vi "Func_SpecificTagReferences.vi"(8 "error in (no error)":errorcluster, 10 "Paths Array":path[](array[path]), 11 "Data Type Name":string) -> (0 "error out":errorcluster)   [LabVIEW 2010, in "TemplateGenerator.lvlib"]
uses:
  TemplateGenerator.lvlib
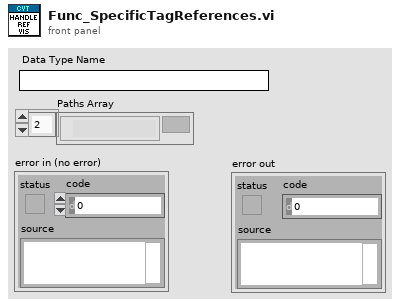
[diagram p1: front panel]
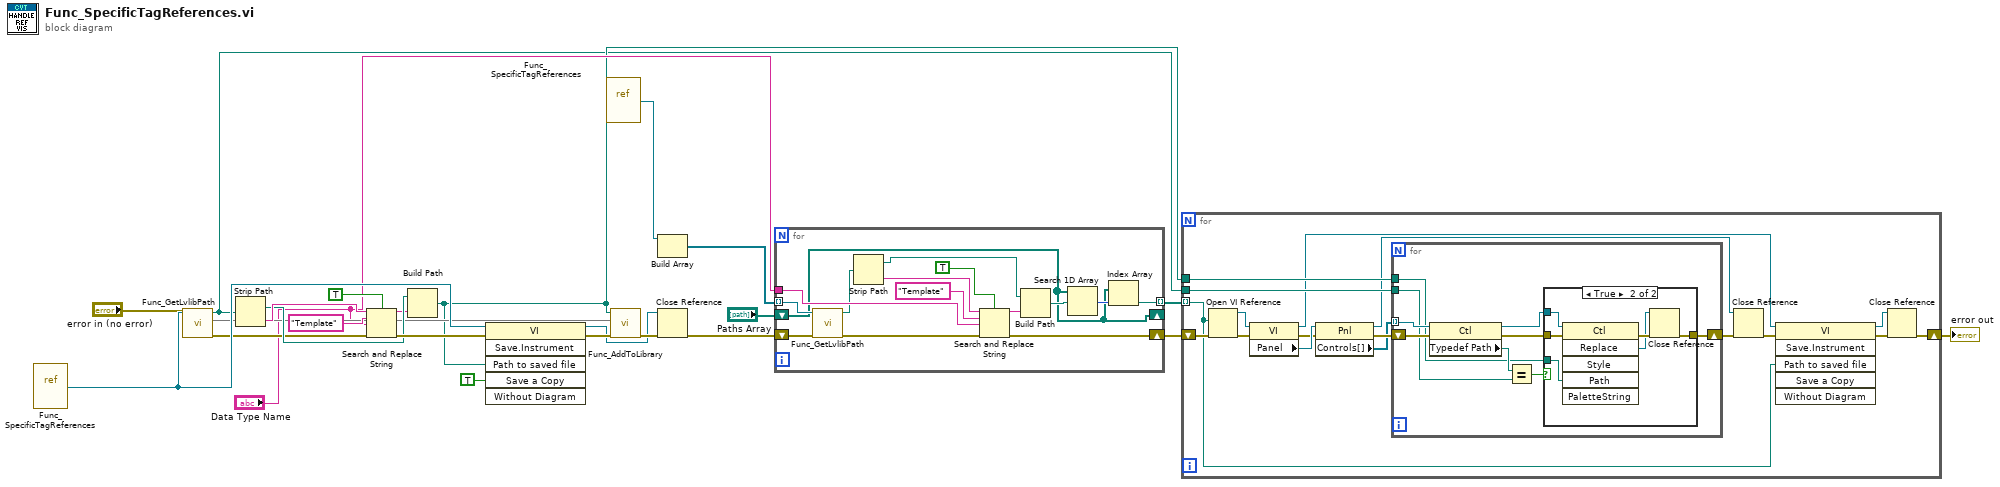
[diagram p0: block diagram]
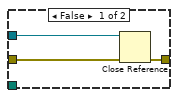
[diagram p2: hidden frame]
diagram:
  n1 = vi-ref "Func_SpecificTagReferences.vi"() -> (w19:refnum<vi>)
  n2 = call "Func_GetLvlibPath.vi"("error in (no error)"="error in (no error)", "VI in"=w19) -> ("error out"=w16:errorcluster, 2:w17, "VI Path"=w3:path)  [unwired: 7 in]
  n3 = Strip Path(path=w3) -> (stripped path=w22:path, name=w26:string)
  n4 = Search and Replace String(case sensitive?=TRUE ("ignore case? (F)"), input string=w26, search string="Template", replace string="Data Type Name", error in=w16) -> (result string=w21:string, error out=w24:errorcluster)  [unwired: 3 in, 2 out]
  n5 = Build Path(base path=w22, name or relative path=w21) -> (appended path=w4:path)
  n6 = invoke class="VI" method="Save.Instrument"(reference=w19, error in=w24, "Path to saved file"=w4, "Save a Copy"=TRUE) -> (reference out=w11:refnum<vi>, error out=w18:errorcluster)  [unwired: 2 in, 4 out]
  n7 = vi-ref "Func_SpecificTagReferences.vi"() -> (w13:refnum<vi>)
  n8 = call "Func_AddToLibrary.vi"("error in (no error)"=w18, "Library Path"=w17, "VI Path"=w4) -> ("error out"=w12:errorcluster)  [unwired: 8 in]
  n9 = Build Array(w13) -> (w10:refnum<vi>[], w14:refnum<vi>, w15:refnum<vi>)
  n10 = Close Reference(reference=w11, error in (no error)=w12) -> (error out=w9:errorcluster)
  n11 = for {
    tunnel: w10 -> [w40] mode=indexing
    shift-right: [w32] -> w5
    shift-left: w9 -> [w41]
    tunnel: "Data Type Name" -> [w34]
    shift-right: [w28] -> _
    shift-left: "Paths Array" -> [w28]
    tunnel: [w27] -> w6 mode=indexing
    n12 = call "Func_GetLvlibPath.vi"("error in (no error)"=w41, "VI in"=w40) -> ("error out"=w31:errorcluster, "VI Path"=w33:path)  [unwired: 8 in]
    n13 = Strip Path(path=w33) -> (stripped path=w38:path, name=w35:string)
    n14 = Search and Replace String(case sensitive?=TRUE ("ignore case? (F)"), input string=w35, search string="Template", replace string=w34, error in=w31) -> (result string=w39:string, error out=w32:errorcluster)  [unwired: 3 in, 2 out]
    n15 = Build Path(base path=w38, name or relative path=w39) -> (appended path=w30:path)
    n16 = Search 1D Array(1D array=w28, element=w30) -> (index of element=w29:i32)  [unwired: 1 in]
    n17 = Index Array(array=w28, index=w29) -> (element=w27:path)
  }
  n18 = for {
    tunnel: w6 -> [w43] mode=indexing
    shift-right: [w42] -> w2
    shift-left: w5 -> [w58]
    tunnel: w4 -> [w50]
    tunnel: w3 -> [w51]
    n19 = Open VI Reference(vi path=w43, error in (no error)=w58) -> (vi reference=w57:refnum<vi>, error out=w56:errorcluster)  [unwired: 4 in]
    n20 = property class="VI"(reference=w57, error in=w56) -> (reference out=w45:refnum<vi>, error out=w54:errorcluster, "Panel"=w55:refnum<vi>)
    n21 = property class="Pnl"(reference=w55, error in=w54) -> (reference out=w48:refnum<vi>, error out=w53:errorcluster, "Controls[]"=w52:refnum<vi>[])
    n22 = for {
      shift-right: [w61] -> w49
      shift-left: w53 -> [w67]
      tunnel: w52 -> [w66] mode=indexing
      tunnel: w51 -> [w64]
      tunnel: w50 -> [w59]
      n23 = property class="Ctl"(reference=w66, error in=w67) -> (reference out=w60:refnum<vi>, error out=w62:errorcluster, "Typedef Path"=w65:path)
      n24 = Equal?(x=w65, y=w64) -> (x = y?=w63:bool)
      n25 = case shown="True" w63 {
        tunnel: w62 -> [w70 w76]
        tunnel: [w69 w71] -> w61
        tunnel: w60 -> [w68 w75]
        tunnel: w59 -> [_ w74]
        frame False {
          n26 = Close Reference(reference=w68, error in (no error)=w70) -> (error out=w69:errorcluster)
        }
        frame True {
          n27 = invoke class="Ctl" method="Replace"(reference=w75, error in=w76, "Path"=w74) -> (error out=w73:errorcluster, "Replace"=w72:refnum<vi>)  [unwired: 3 in, 4 out]
          n28 = Close Reference(reference=w72, error in (no error)=w73) -> (error out=w71:errorcluster)
        }
      }
    }
    n29 = Close Reference(reference=w48, error in (no error)=w49) -> (error out=w47:errorcluster)
    n30 = invoke class="VI" method="Save.Instrument"(reference=w45, error in=w47, "Path to saved file"=w43) -> (reference out=w44:refnum<vi>, error out=w46:errorcluster)  [unwired: 3 in, 4 out]
    n31 = Close Reference(reference=w44, error in (no error)=w46) -> (error out=w42:errorcluster)
  }
  "error out" <- w2
